vi "TakeVoltageMeasurementWritetoFile.vi"   [LabVIEW 2009]
types:
  T1 = enum16{"open", "replace", "create", "open or create", "replace or create", "replace or create with confirmation"}
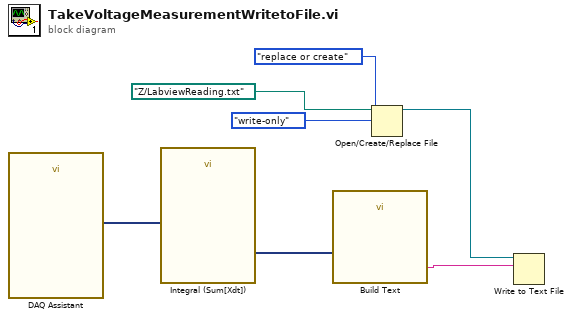
[diagram p0: block diagram]
diagram:
  n1 = call "DAQ Assistant"() -> ("data"=w7:dynamicdata)  [unwired: 17 in, 2 out]
  n2 = call "Integral (Sum[Xdt])"("Signals"=w7) -> ("Result"=w6:dynamicdata)  [unwired: 5 in, 1 out]
  n3 = call "Build Text"("VoltageAverage"=w6) -> ("Result"=w5:string)  [unwired: 13 in, 1 out]
  n4 = Open/Create/Replace File(file path (use dialog)=path "Z:/LabviewReading.txt", operation (0:open)=T1."replace or create", access (0:read/write)=enum16{"read/write", "read-only", "write-only"}."write-only") -> (refnum out=w4:refnum<file>)  [unwired: 3 in, 2 out]
  n5 = Write to Text File(file (use dialog)=w4, text=w5) -> ()  [unwired: 2 in, 3 out]
